vi "TDMSRowSelect.vi"(6 "Digital Out Tasks":tag[](array[tag])=["PXI1Slot2/port0", "PXI1Slot3/port0", "PXI1Slot6/port0"], 7 "Group Name":string, 8 "Error In":errorcluster, 10 "BitMaskValues in":u32[][](array[numeric]), 11 "tdms file In":refnum<k34>) -> (0 "Error Out":errorcluster)   [LabVIEW 2011]
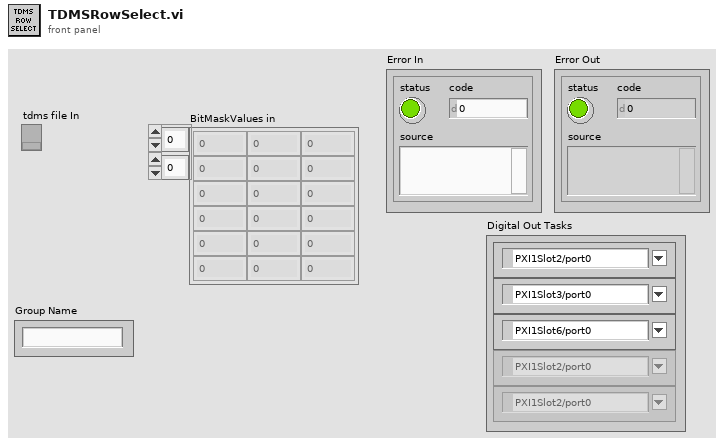
[diagram p1: front panel]
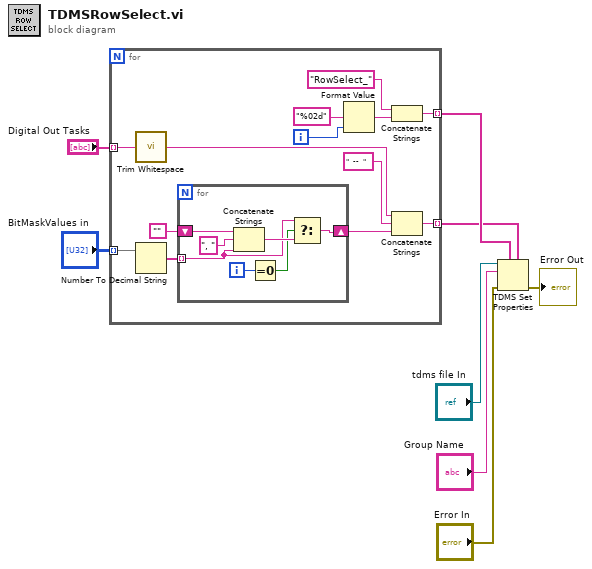
[diagram p0: block diagram]
diagram:
  n1 = for {
    tunnel: "Digital Out Tasks" -> [w21] mode=indexing
    tunnel: "BitMaskValues in" -> [w20] mode=indexing
    tunnel: [w16] -> w4 mode=indexing
    tunnel: [w9] -> w3 mode=indexing
    i -> [w15]
    n2 = call <vilib>:"Trim Whitespace.vi"("string"=w21) -> ("trimmed string"=w12:string)  [unwired: 1 in]
    n3 = Number To Decimal String(number=w20) -> (decimal integer string=w18:string[])  [unwired: 1 in]
    n4 = for {
      tunnel: w18 -> [w22] mode=indexing
      shift-right: [w26] -> w10
      shift-left: "" -> [w28]
      i -> [w24]
      n5 = Concatenate Strings(w28, ", " ("string"), w22) -> (w25:string)
      n6 = Equal To 0?(x=w24) -> (x = 0?=w23:bool)
      n7 = Select(t=w22, s=w23, f=w25) -> (s? t:f=w26:string)
    }
    n8 = Format Value(format string="%02d", value (0)=w15) -> (output string=w13:string)  [unwired: 1 in]
    n9 = Concatenate Strings("RowSelect_" ("string"), w13) -> (w16:string)
    n10 = Concatenate Strings(w12, "  --  " ("string"), w10) -> (w9:string)
  }
  n11 = TDMS Set Properties(5:w3, 7:w4, 8:"Error In", 10:"Group Name", 11:"tdms file In") -> (0:→"Error Out":errorcluster)  [unwired: 1 in, 3 out]
